vi "lua_rawseti.vi"(8 "error in (no error)":errorcluster, 9 "n":i64, 10 "index":i32, 11 "lua_state_p":u64) -> (0 "error out":errorcluster, 3 "lua_state_p out":u64)   [LabVIEW 2020, in "lua.dll.lvlib"]
doc: "Does the equivalent of t[n] = v, where t is the value at the given valid index and v is the value at the top of the stack.\n\nThis function pops the value from the stack. The assignment is raw; that is, it does not invoke metamethods."
uses:
  lua.dll.lvlib
  lua54.dll
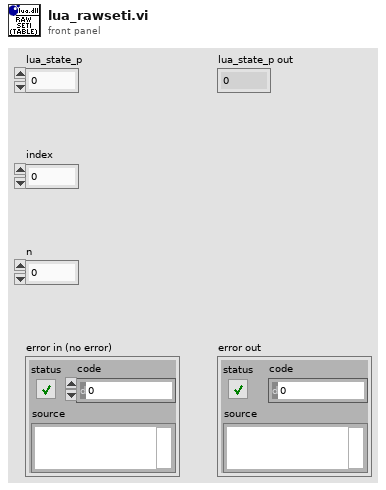
[diagram p1: front panel]
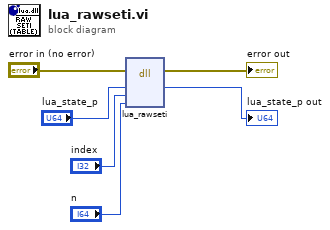
[diagram p0: block diagram]
diagram:
  n1 = dll-call lib="C:/Users/Nicholas Folse/Documents/workspace/github-tauterra.llc/Lua for LabVIEW/lib/lua.dll/lua54**.*" fn="lua_rawseti"(error in="error in (no error)", "lua_state_p"="lua_state_p", "index"="index", "n"="n") -> (error out=→"error out":errorcluster, "lua_state_p"=→"lua_state_p out":u64)  [unwired: 5 in, 1 out]
